vi "Copy Package.vi"(8 "error in (no error)":errorcluster, 11 "PostBuildSupport in":refnum<class "PostBuildSupport.lvclass">) -> (0 "error out":errorcluster, 3 "PostBuildSupport out":refnum<class "PostBuildSupport.lvclass">)   [LabVIEW 2016, in "PostBuildSupport.lvclass"]
uses:
  PostBuildSupport.lvclass
  PostBuildSupport.lvclass/PostBuildSupport.ctl
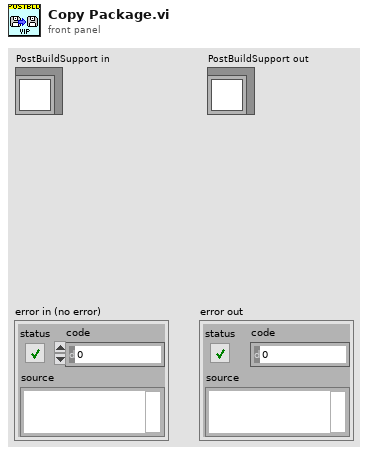
[diagram p1: front panel]
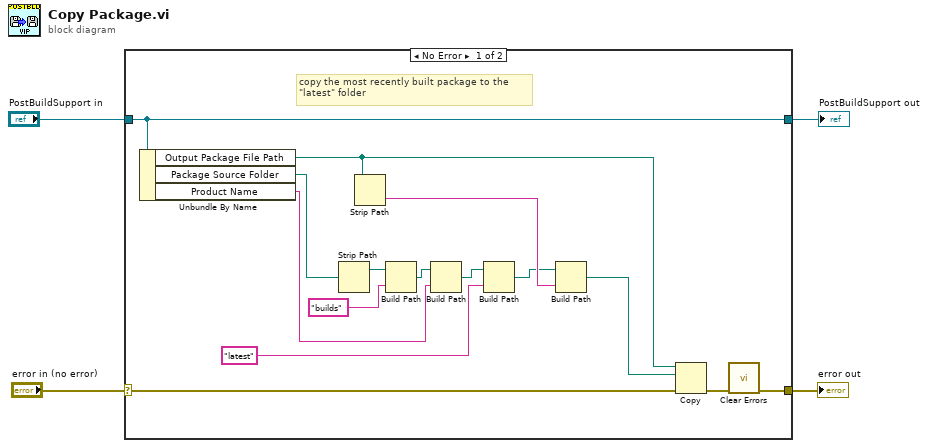
[diagram p0: block diagram]
diagram:
  n1 = case shown="No Error" "error in (no error)" {
    selector: "error in (no error)" -> [w8 w21]
    tunnel: [w5 w21] -> w4
    tunnel: "PostBuildSupport in" -> [w7 w20]
    tunnel: [w7 w20] -> w1
    frame No Error {
      # "copy the most recently built package to the \n\"latest\" folder"
      n2 = Unbundle By Name(w7) -> ("Output Package File Path"=w9:path, "Package Source Folder"=w11:path, "Product Name"=w10:string)
      n3 = Strip Path(path=w11) -> (stripped path=w19:path)  [unwired: 1 out]
      n4 = Strip Path(path=w9) -> (name=w18:string)  [unwired: 1 out]
      n5 = Build Path(base path=w19, name or relative path="builds") -> (appended path=w15:path)
      n6 = Build Path(base path=w15, name or relative path=w10) -> (appended path=w14:path)
      n7 = Build Path(base path=w14, name or relative path="latest") -> (appended path=w12:path)
      n8 = Build Path(base path=w12, name or relative path=w18) -> (appended path=w17:path)
      n9 = Copy(8:w8, 10:w17, 11:w9) -> (0:w6:errorcluster)  [unwired: 2 in, 2 out]
      n10 = call <vilib>:"Clear Errors.vi"("error in (no error)"=w6) -> ("error out"=w5:errorcluster)  [unwired: 5 in, 1 out]
    }
    frame Error {
    }
  }
  "error out" <- w4
  "PostBuildSupport out" <- w1
